vi "Robot Global Data.vi"() -> ()   [LabVIEW 2020]
doc: "This global VI can contain as many global variables as you need. To create a global variable, place a control on the panel, give it a good name. To read or write to it from a VI, drag the icon to the diagram of that VI. You can also drag from the project. Click on the node to change which global you access. You shouldn't have multiple locations writing to a global or it will cause a race-condition."
uses:
  <vilib>/Rock Robotics/WPI/Camera/WPI_CameraImageSize.ctl
  <vilib>/Rock Robotics/WPI/DriverStation/WPI_DriverStationRobotMode2.ctl
panel:
  in  "Transfer Release Setpoint":dbl
  in  "Transfer Up Setpoint":dbl
  in  "Intake Setpoint":dbl
  in  "Shooter Setpoint":dbl
  in  "Auto Pick":string="record"
  in  "Auto List":string="record"
  in  "Record Path":bool
  in  "Wheel":dbl min=-1.0 max=1.0 step=1e-05 format="%_8g"
  in  "Throtle":dbl min=-1.0 max=1.0 step=1e-05 format="%_8g"
  in  "Climb Traversal":bool
  in  "Transfer Release":bool
  in  "Transfer Up":bool
  in  "Climb Hook":bool
  in  "Intake Arm":bool
  in  "Intake":bool
  in  "Shooter":bool
  in  "Robot Mode":T1
  in  "image size":T2=enum."320x240"
  in  "Enable Vision":bool
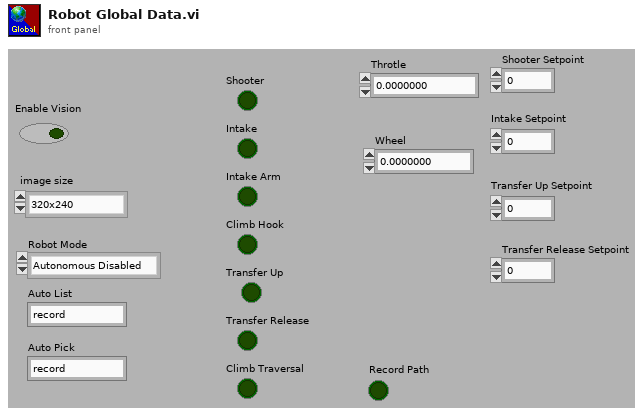
[diagram p1: front panel]
types:
  T1 = typedef "WPI_DriverStationRobotMode2.ctl" = enum16{"Autonomous Disabled", "Autonomous Enabled", "Teleop Disabled", "Teleop Enabled", "Disconnected", "Finish", "Test Disabled", "Test Enabled", "Emergency Stopped"}
  T2 = typedef "WPI_CameraImageSize.ctl" = enum16{"640x480", "320x240", "160x120", "Custom"}
diagram:
